vi "Clustering----.vi"() -> ()   [LabVIEW 2020]
panel:
  out "appended array":cluster{"array":dbl[], "array":dbl[]}[](array[cluster])
  in  "stop":bool
  out "byte swapped":u16
  out "Azimuth":u32
  out "100bytes":string
  out "Azimuth2":dbl
  out "substring 2":string
  in  "channel 1":bool=TRUE
  in  "channel 0":bool
  in  "channel 2":bool
  in  "channel 3":bool
  in  "channel 4":bool
  in  "channel 5":bool=TRUE
  in  "channel 6":bool
  in  "channel 7":bool
  in  "channel 8":bool
  in  "channel 9":bool
  in  "channel 10":bool
  in  "channel 11":bool
  in  "channel 12":bool
  in  "channel 13":bool
  in  "channel 14":bool
  in  "channel 15":bool
  in  "점 개수":i32
  out "Mixed Signal Graph":cluster{"array":dbl[], "array":dbl[]}[](graph)
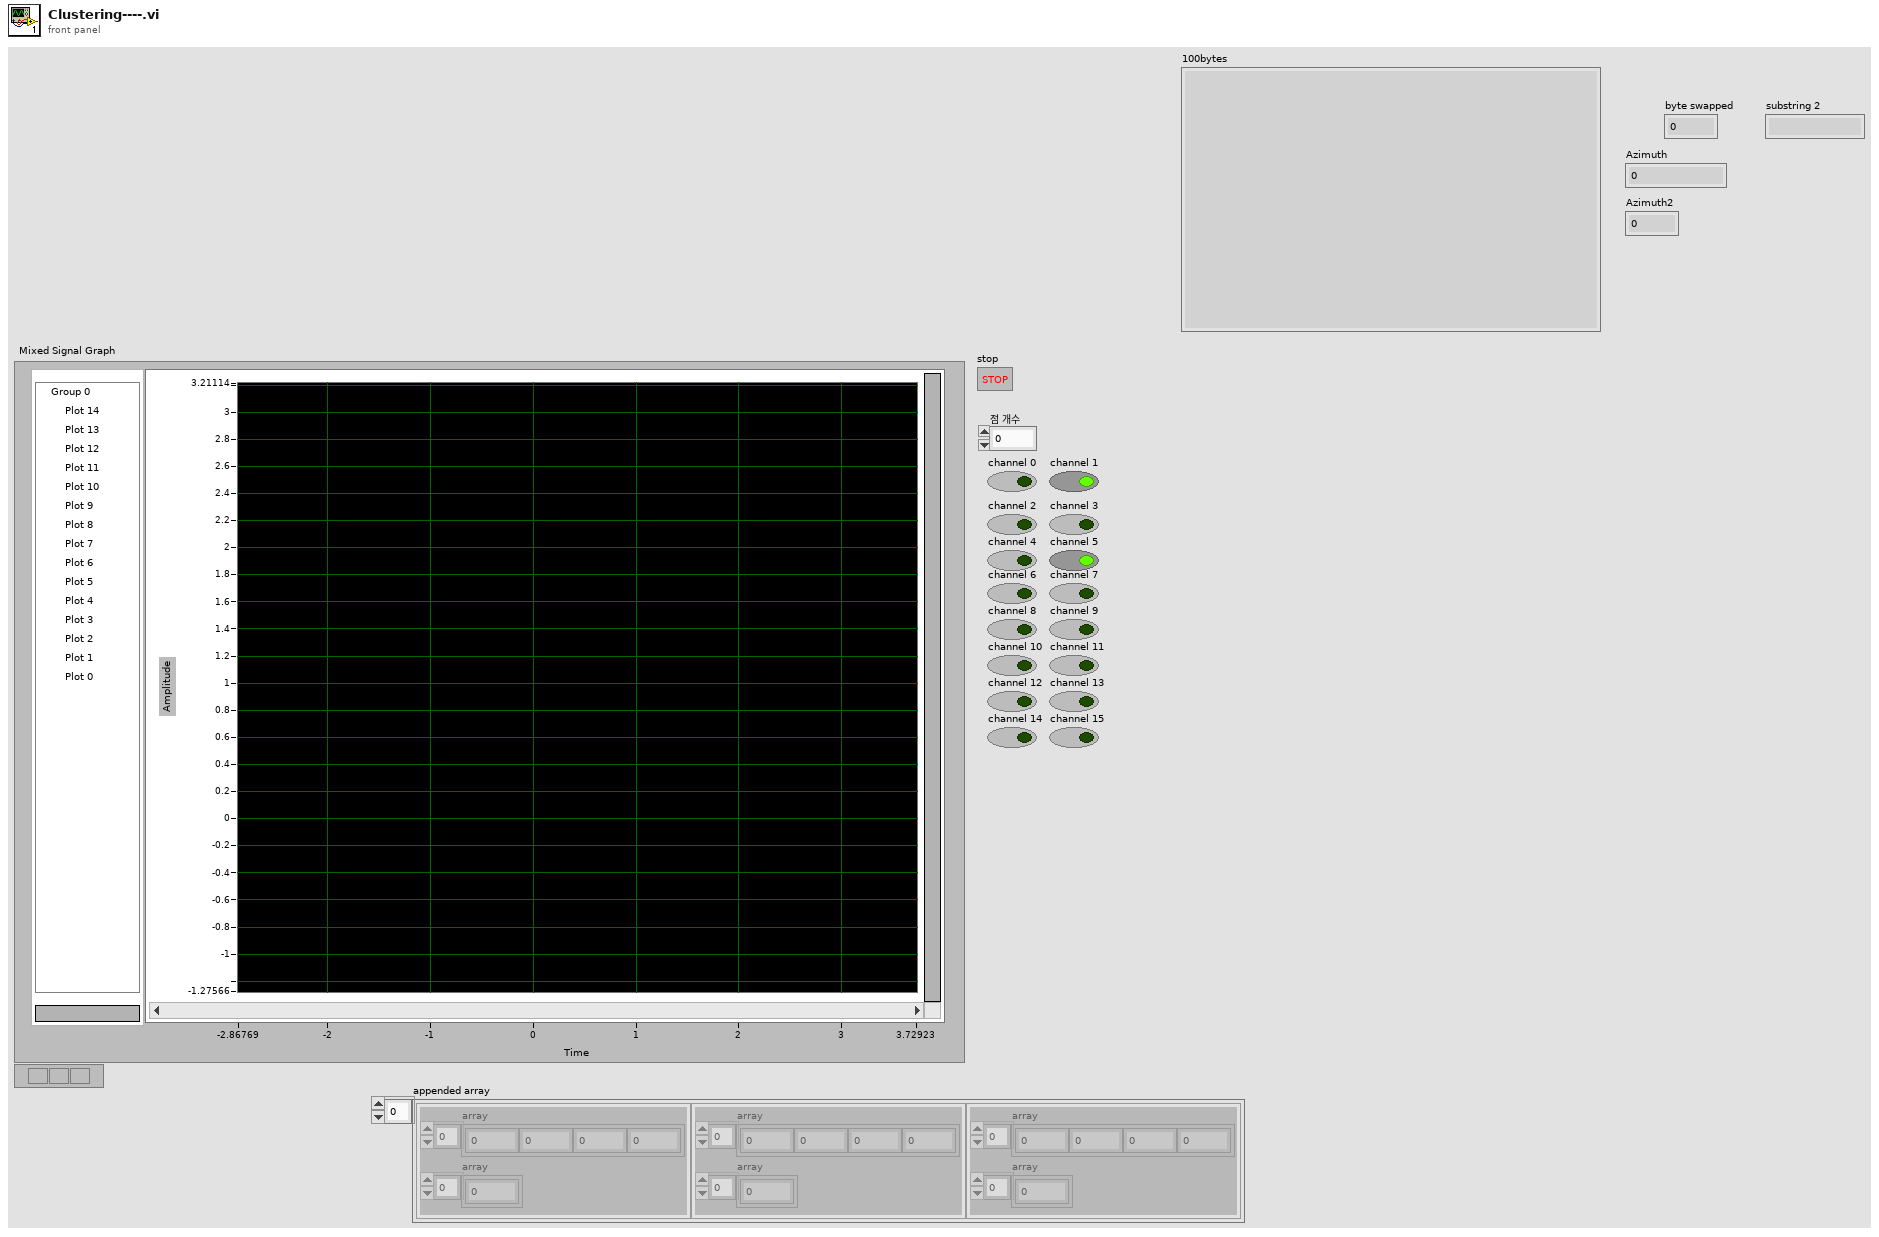
[diagram p1: front panel]
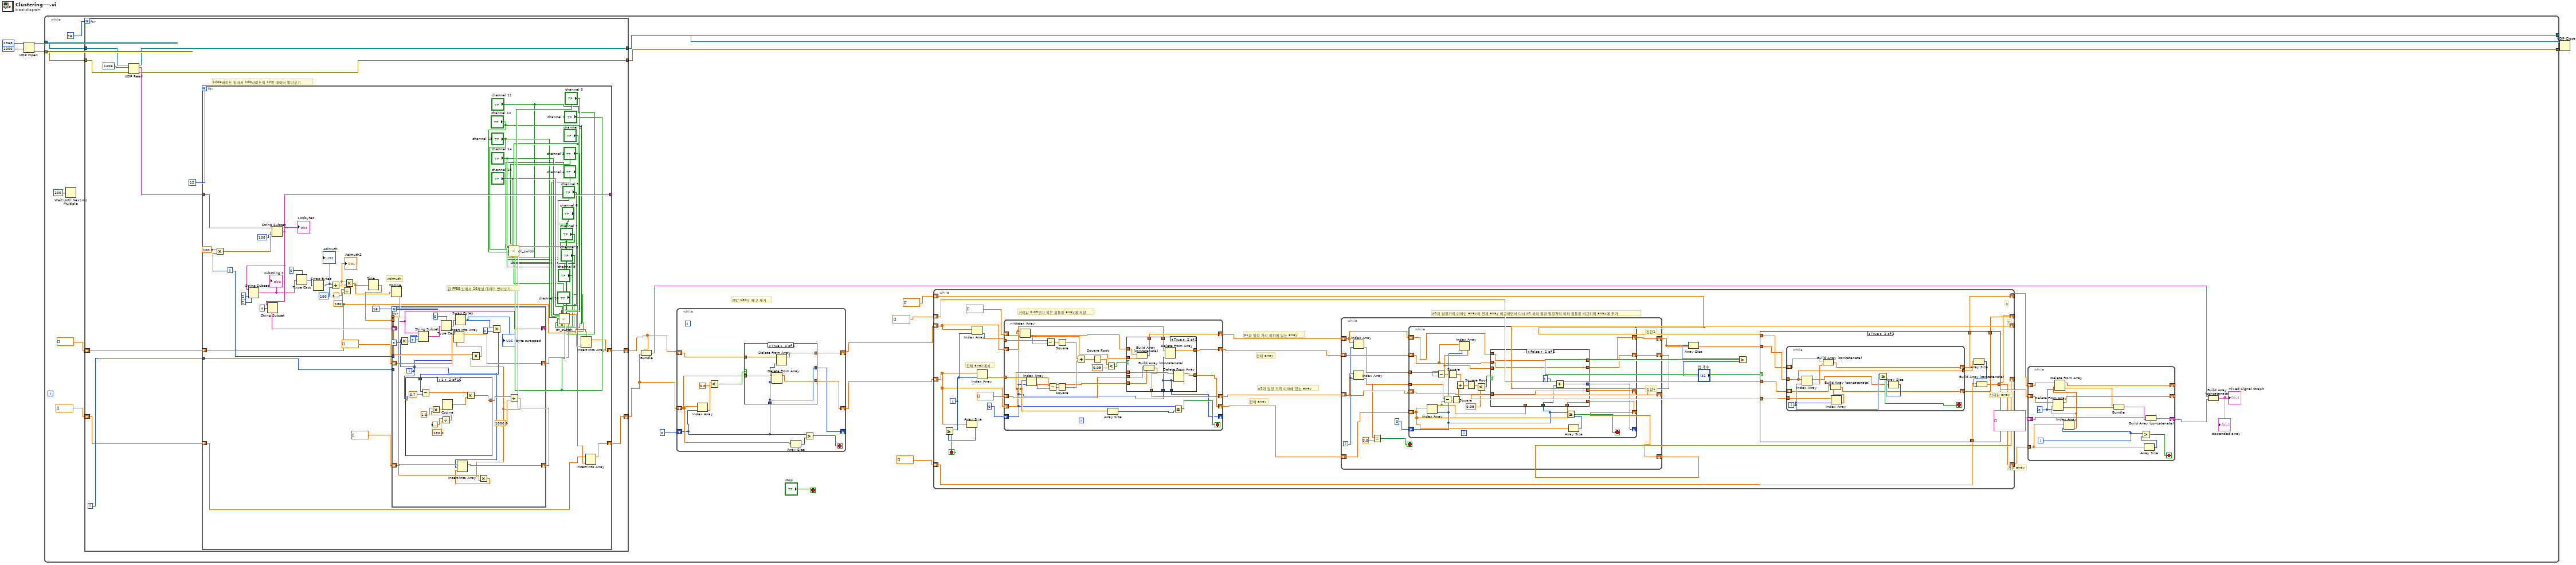
[diagram p0: block diagram]
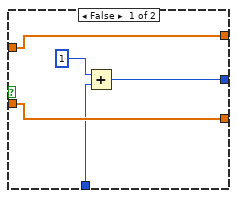
[diagram p2: hidden frame]
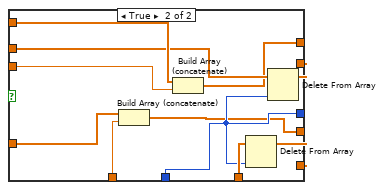
[diagram p4: hidden frame]
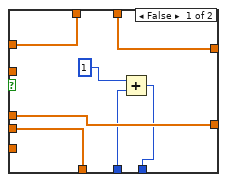
[diagram p5: hidden frame]
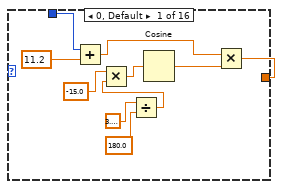
[diagram p6: hidden frame]
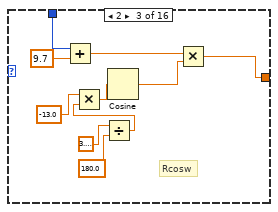
[diagram p7: hidden frame]
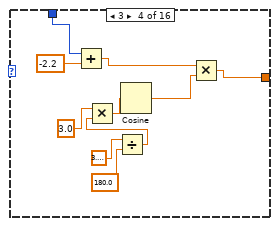
[diagram p8: hidden frame]
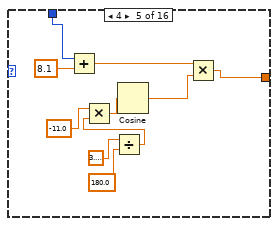
[diagram p9: hidden frame]
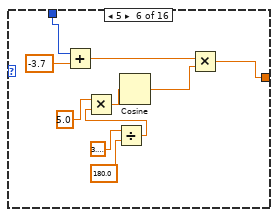
[diagram p10: hidden frame]
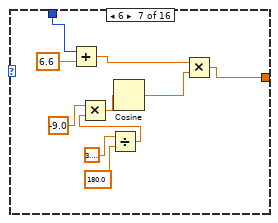
[diagram p11: hidden frame]
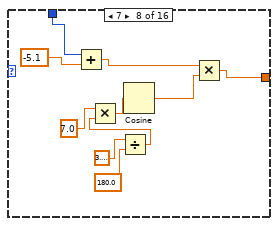
[diagram p12: hidden frame]
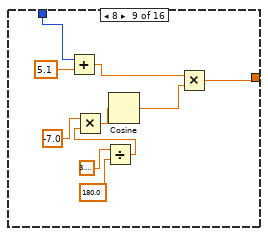
[diagram p13: hidden frame]
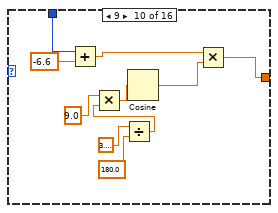
[diagram p14: hidden frame]
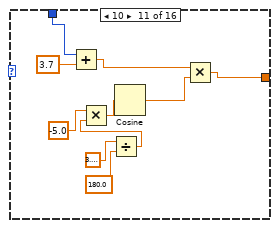
[diagram p15: hidden frame]
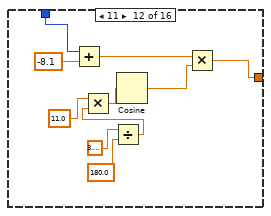
[diagram p16: hidden frame]
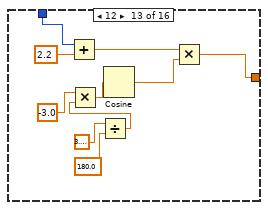
[diagram p17: hidden frame]
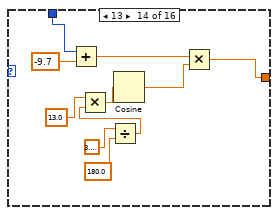
[diagram p18: hidden frame]
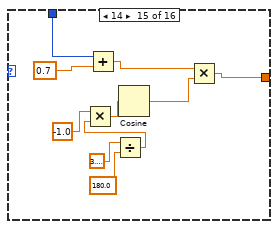
[diagram p19: hidden frame]
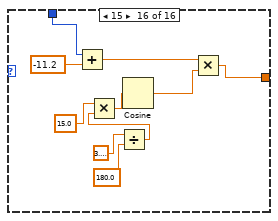
[diagram p20: hidden frame]
diagram:
  n1 = UDP Open(9:1000 ("timeout ms (25000)"), 11:u16 2368 ("port")) -> (port=w3:refnum<k16>, 0:w4:errorcluster)  [unwired: 3 in, 1 out]
  n2 = while {
    tunnel: w4 -> [w29]
    tunnel: w3 -> [w28]
    tunnel: [w27] -> w2
    tunnel: [w26] -> w1
    stop <- "stop" stop-if-true
    # "개수 array"
    # "Y"
    # "X"
    # "삭제된 array"
    # "전방 180도 빼고 제거"
    n3 = Wait Until Next ms Multiple(millisecond multiple=u32 100) -> ()  [unwired: 1 out]
    n4 = for {
      N: 76 -> [_]
      shift-right: [w218] -> w9
      shift-left: dbl[] [] ("array") -> [w216]
      shift-right: [w219] -> w10
      shift-left: dbl[] [] ("array") -> [w217]
      tunnel: w28 -> [w225]
      tunnel: [w222] -> w27
      tunnel: w29 -> [w226]
      tunnel: [w221] -> w26
      i -> [w220]
      # "1206바이트 읽어서 100바이트씩 12번 데이터 받아오기"
      n5 = UDP Read(connection ID=w225, max size (548)=1206, 8:w226) -> (data out=w224:string, error out=w221:errorcluster, 3:w222:refnum<k16>)  [unwired: 1 in, 2 out]
      n6 = for {
        N: 12 -> [_]
        shift-right: [w243] -> w218
        shift-left: w216 -> [w244]
        shift-right: [w246] -> w219
        shift-left: w217 -> [w248]
        tunnel: w220 -> [w255]
        tunnel: w224 -> [w263]
        tunnel: [w258] -> _
        i -> [w254]
        # "Azimuth"
        # "한 FFEE 안에서 16채널 데이터 받아오기"
        n7 = Multiply(x=100.0, y=w254) -> (x*y=w261:dbl)
        n8 = String Subset(string=w263, offset (0)=w261, length (rest)=100 ("length (rest)")) -> (substring=w258:string)
        "100bytes" <- w258
        n9 = String Subset(string=w258, offset (0)=2, length (rest)=2 ("length (rest)")) -> (substring=w257:string)
        "substring 2" <- w257
        n10 = String Subset(string=w258, offset (0)=4) -> (substring=w260:string)  [unwired: 1 in]
        n11 = Type Cast(type=u16 0, x=w257) -> (*(type *) &x=w256:u16)
        n12 = Swap Bytes(anything=w256) -> (byte swapped=w273:u16)
        "Azimuth" <- w273
        n13 = Divide(x=w273, y=u32 100) -> (x/y=w271:dbl)
        "Azimuth2" <- w271
        n14 = Divide(x=3.141592653589793, y=180.0) -> (x/y=w268:dbl)
        n15 = Multiply(x=w271, y=w268) -> (x*y=w266:dbl)
        n16 = Sine(x=w266) -> (sin(x)=w267:dbl)
        n17 = Cosine(x=w266) -> (cos(x)=w265:dbl)
        n18 = for {
          N: 16 -> [_]
          shift-right: [w295] -> w251
          shift-left: dbl[] [] ("array") -> [w296]
          tunnel: w267 -> [w289]
          shift-right: [w290] -> w253
          shift-left: dbl[] [] ("array") -> [w291]
          tunnel: w265 -> [w288]
          shift-right: [w283] -> _
          shift-left: w260 -> [w283]
          tunnel: w254 -> [_]
          tunnel: w255 -> [_]
          i -> [w278]
          n19 = Multiply(x=w278, y=3) -> (x*y=w297:i32)
          n20 = String Subset(string=w283, offset (0)=w297, length (rest)=2 ("length (rest)")) -> (substring=w285:string)
          n21 = Type Cast(type=u16 0, x=w285) -> (*(type *) &x=w284:u16)
          n22 = Swap Bytes(anything=w284) -> (byte swapped=w279:u16)
          "byte swapped" <- w279
          n23 = Multiply(x=w279, y=u32 2) -> (x*y=w293:u32)
          n24 = case shown="1" w278 {
            tunnel: w293 -> [w302 w312 w322 w331 w341 w351 w361 w371 w381 w391 w401 w411 w421 w431 w441 w451]
            tunnel: [w308 w313 w323 w333 w343 w353 w363 w373 w383 w393 w403 w413 w423 w433 w443 w453] -> w282
            frame 0, Default {
              n25 = Add(x=w302, y=11.2) -> (x+y=w300:dbl)
              n26 = Divide(x=3.141592653589793, y=180.0) -> (x/y=w303:dbl)
              n27 = Multiply(x=-15.0 ("y"), y=w303) -> (x*y=w304:dbl)
              n28 = Cosine(x=w304) -> (cos(x)=w309:dbl)
              n29 = Multiply(x=w300, y=w309) -> (x*y=w308:dbl)
            }
            frame 1 {
              n30 = Subtract(x=w312, y=0.7) -> (x-y=w310:dbl)
              n31 = Divide(x=3.141592653589793, y=180.0) -> (x/y=w315:dbl)
              n32 = Multiply(x=1.0 ("y"), y=w315) -> (x*y=w316:dbl)
              n33 = Cosine(x=w316) -> (cos(x)=w314:dbl)
              n34 = Multiply(x=w310, y=w314) -> (x*y=w313:dbl)
            }
            frame 2 {
              # "Rcosw"
              n35 = Add(x=w322, y=9.7) -> (x+y=w320:dbl)
              n36 = Divide(x=3.141592653589793, y=180.0) -> (x/y=w325:dbl)
              n37 = Multiply(x=-13.0 ("y"), y=w325) -> (x*y=w326:dbl)
              n38 = Cosine(x=w326) -> (cos(x)=w324:dbl)
              n39 = Multiply(x=w320, y=w324) -> (x*y=w323:dbl)
            }
            frame 3 {
              n40 = Add(x=w331, y=-2.2) -> (x+y=w330:dbl)
              n41 = Divide(x=3.141592653589793, y=180.0) -> (x/y=w335:dbl)
              n42 = Multiply(x=3.0 ("y"), y=w335) -> (x*y=w336:dbl)
              n43 = Cosine(x=w336) -> (cos(x)=w334:dbl)
              n44 = Multiply(x=w330, y=w334) -> (x*y=w333:dbl)
            }
            frame 4 {
              n45 = Add(x=w341, y=8.1) -> (x+y=w340:dbl)
              n46 = Divide(x=3.141592653589793, y=180.0) -> (x/y=w345:dbl)
              n47 = Multiply(x=-11.0 ("y"), y=w345) -> (x*y=w346:dbl)
              n48 = Cosine(x=w346) -> (cos(x)=w344:dbl)
              n49 = Multiply(x=w340, y=w344) -> (x*y=w343:dbl)
            }
            frame 5 {
              n50 = Add(x=w351, y=-3.7) -> (x+y=w350:dbl)
              n51 = Divide(x=3.141592653589793, y=180.0) -> (x/y=w355:dbl)
              n52 = Multiply(x=5.0 ("y"), y=w355) -> (x*y=w356:dbl)
              n53 = Cosine(x=w356) -> (cos(x)=w354:dbl)
              n54 = Multiply(x=w350, y=w354) -> (x*y=w353:dbl)
            }
            frame 6 {
              n55 = Add(x=w361, y=6.6) -> (x+y=w360:dbl)
              n56 = Divide(x=3.141592653589793, y=180.0) -> (x/y=w365:dbl)
              n57 = Multiply(x=-9.0 ("y"), y=w365) -> (x*y=w366:dbl)
              n58 = Cosine(x=w366) -> (cos(x)=w364:dbl)
              n59 = Multiply(x=w360, y=w364) -> (x*y=w363:dbl)
            }
            frame 7 {
              n60 = Add(x=w371, y=-5.1) -> (x+y=w370:dbl)
              n61 = Divide(x=3.141592653589793, y=180.0) -> (x/y=w375:dbl)
              n62 = Multiply(x=7.0 ("y"), y=w375) -> (x*y=w376:dbl)
              n63 = Cosine(x=w376) -> (cos(x)=w374:dbl)
              n64 = Multiply(x=w370, y=w374) -> (x*y=w373:dbl)
            }
            frame 8 {
              n65 = Add(x=w381, y=5.1) -> (x+y=w380:dbl)
              n66 = Divide(x=3.141592653589793, y=180.0) -> (x/y=w385:dbl)
              n67 = Multiply(x=-7.0 ("y"), y=w385) -> (x*y=w386:dbl)
              n68 = Cosine(x=w386) -> (cos(x)=w384:dbl)
              n69 = Multiply(x=w380, y=w384) -> (x*y=w383:dbl)
            }
            frame 9 {
              n70 = Add(x=w391, y=-6.6) -> (x+y=w390:dbl)
              n71 = Divide(x=3.141592653589793, y=180.0) -> (x/y=w395:dbl)
              n72 = Multiply(x=9.0 ("y"), y=w395) -> (x*y=w396:dbl)
              n73 = Cosine(x=w396) -> (cos(x)=w394:dbl)
              n74 = Multiply(x=w390, y=w394) -> (x*y=w393:dbl)
            }
            frame 10 {
              n75 = Add(x=w401, y=3.7) -> (x+y=w400:dbl)
              n76 = Divide(x=3.141592653589793, y=180.0) -> (x/y=w405:dbl)
              n77 = Multiply(x=-5.0 ("y"), y=w405) -> (x*y=w406:dbl)
              n78 = Cosine(x=w406) -> (cos(x)=w404:dbl)
              n79 = Multiply(x=w400, y=w404) -> (x*y=w403:dbl)
            }
            frame 11 {
              n80 = Add(x=w411, y=-8.1) -> (x+y=w410:dbl)
              n81 = Divide(x=3.141592653589793, y=180.0) -> (x/y=w415:dbl)
              n82 = Multiply(x=11.0 ("y"), y=w415) -> (x*y=w416:dbl)
              n83 = Cosine(x=w416) -> (cos(x)=w414:dbl)
              n84 = Multiply(x=w410, y=w414) -> (x*y=w413:dbl)
            }
            frame 12 {
              n85 = Add(x=w421, y=2.2) -> (x+y=w420:dbl)
              n86 = Divide(x=3.141592653589793, y=180.0) -> (x/y=w425:dbl)
              n87 = Multiply(x=-3.0 ("y"), y=w425) -> (x*y=w426:dbl)
              n88 = Cosine(x=w426) -> (cos(x)=w424:dbl)
              n89 = Multiply(x=w420, y=w424) -> (x*y=w423:dbl)
            }
            frame 13 {
              n90 = Add(x=w431, y=-9.7) -> (x+y=w430:dbl)
              n91 = Divide(x=3.141592653589793, y=180.0) -> (x/y=w435:dbl)
              n92 = Multiply(x=13.0 ("y"), y=w435) -> (x*y=w436:dbl)
              n93 = Cosine(x=w436) -> (cos(x)=w434:dbl)
              n94 = Multiply(x=w430, y=w434) -> (x*y=w433:dbl)
            }
            frame 14 {
              n95 = Add(x=w441, y=0.7) -> (x+y=w440:dbl)
              n96 = Divide(x=3.141592653589793, y=180.0) -> (x/y=w445:dbl)
              n97 = Multiply(x=-1.0 ("y"), y=w445) -> (x*y=w446:dbl)
              n98 = Cosine(x=w446) -> (cos(x)=w444:dbl)
              n99 = Multiply(x=w440, y=w444) -> (x*y=w443:dbl)
            }
            frame 15 {
              n100 = Add(x=w451, y=-11.2) -> (x+y=w450:dbl)
              n101 = Divide(x=3.141592653589793, y=180.0) -> (x/y=w455:dbl)
              n102 = Multiply(x=15.0 ("y"), y=w455) -> (x*y=w456:dbl)
              n103 = Cosine(x=w456) -> (cos(x)=w454:dbl)
              n104 = Multiply(x=w450, y=w454) -> (x*y=w453:dbl)
            }
          }
          n105 = Divide(x=w282, y=1000.0) -> (x/y=w280:dbl)
          n106 = Multiply(x=w289, y=w280) -> (x*y=w292:dbl)
          n107 = Insert Into Array(array=w296, index=w278, new element=w292) -> (w295:dbl[])
          n108 = Multiply(x=w280, y=w288) -> (x*y=w287:dbl)
          n109 = Insert Into Array(array=w291, index=w278, new element=w287) -> (w290:dbl[])
        }
        n110 = call "ch_switch.vi"("channel 14"="channel 14", "channel 4"="channel 4", "channel 13"="channel 13", "channel 5"="channel 5", "channel 12"="channel 12", "channel 6"="channel 6", "channel 7"="channel 7", "channel 3"="channel 3", "channel 8"="channel 8", "channel 15"="channel 15", "channel 9"="channel 9", "channel 2"="channel 2", "channel 10"="channel 10", "channel 1"="channel 1", "channel 11"="channel 11", "channel 0"="channel 0", "Array in"=w253) -> ("Array out"=w245:dbl[])  [unwired: 10 in]
        n111 = call "ch_switch.vi"("channel 14"="channel 14", "channel 4"="channel 4", "channel 13"="channel 13", "channel 5"="channel 5", "channel 12"="channel 12", "channel 6"="channel 6", "channel 7"="channel 7", "channel 3"="channel 3", "channel 8"="channel 8", "channel 15"="channel 15", "channel 9"="channel 9", "channel 2"="channel 2", "channel 10"="channel 10", "channel 1"="channel 1", "channel 11"="channel 11", "channel 0"="channel 0", "Array in"=w251) -> ("Array out"=w247:dbl[])  [unwired: 10 in]
        n112 = Insert Into Array(array=w248, new element=w247) -> (w246:dbl[])  [unwired: 1 in]
        n113 = Insert Into Array(array=w244, new element=w245) -> (w243:dbl[])  [unwired: 1 in]
      }
    }
    n114 = Bundle("array"=w10, "array"=w9) -> (w11:cluster{"array":dbl[], "array":dbl[]})  [unwired: 1 in]
    n115 = while {
      shift-right: [w51] -> w18
      shift-left: w9 -> [w50]
      shift-right: [w52] -> w22
      shift-left: w10 -> [w53]
      shift-right: [w46] -> _
      shift-left: 0 -> [w47]
      stop <- w48 stop-if-true
      n116 = Index Array(array=w50, index=w47) -> (element=w56:dbl)
      n117 = Less?(x=w56, y=0.0) -> (x < y?=w54:bool)
      n118 = case shown="True" w54 {
        tunnel: w53 -> [w61 w66]
        tunnel: w47 -> [w59 w62]
        tunnel: [w61 w63] -> w52
        tunnel: [w60 w64] -> w51
        tunnel: w50 -> [w60 w65]
        tunnel: [w58 w62] -> w46
        frame False {
          n119 = Add(x=1, y=w59) -> (x+y=w58:i32)
        }
        frame True {
          n120 = Delete From Array(array=w65, index=w62) -> (array with subset deleted=w64:dbl[])  [unwired: 1 in, 1 out]
          n121 = Delete From Array(array=w66, index=w62) -> (array with subset deleted=w63:dbl[])  [unwired: 1 in, 1 out]
        }
      }
      n122 = Array Size(array=w50) -> (size(s)=w49:i32)
      n123 = Greater?(x=w47, y=w49) -> (0:w48:bool)
    }
    n124 = while {
      shift-right: [w73] -> _
      shift-left: w22 -> [w83]
      shift-right: [w77] -> _
      shift-left: w18 -> [w82]
      shift-right: [w74] -> w12
      shift-left: dbl[] [] ("array") -> [w76]
      shift-right: [w70] -> w16
      shift-left: dbl[] [] ("array") -> [w75]
      shift-right: [w68] -> w15
      shift-left: dbl[] [] ("array") -> [w69]
      i -> [w91]
      stop <- w92 stop-if-true
      # "전체 array에서"
      # "전체 array"
      # "p1과 일정 거리 이하에 있는 array"
      # "전체 array"
      # "p1과 일정거리 이하인 array와 전체 array 비교하면서 다시 p1 외의 점과 일정거리 이하 점들을 비교하며 array에 추가"
      # "p1과 일정 거리 이하에 있는 array"
      # "거리값 0.05보다 작은 점들을 array에 저장"
      n125 = Array Size(array=w82) -> (size(s)=w93:i32)
      n126 = Greater Or Equal?(x=w91, y=w93) -> (x >= y?=w92:bool)
      n127 = Index Array(array=w83, index=w91) -> (element=w90:dbl)
      n128 = Index Array(array=w82, index=w91) -> (element=w89:dbl)
      n129 = while {
        tunnel: w90 -> [w197]
        tunnel: w89 -> [w196]
        shift-right: [w182] -> w71
        shift-left: dbl[] [] ("array") -> [w184]
        shift-right: [w183] -> w67
        shift-left: dbl[] [] ("array") -> [w185]
        shift-right: [w179] -> w78
        shift-left: w83 -> [w181]
        shift-right: [w178] -> w72
        shift-left: w82 -> [w180]
        shift-right: [w174] -> _
        shift-left: 0 -> [w175]
        stop <- w176 stop-if-true
        n130 = Index Array(array=w181, index=w175) -> (element=w187:dbl)
        n131 = Index Array(array=w180, index=w175) -> (element=w186:dbl)
        n132 = Subtract(x=w197, y=w187) -> (x-y=w195:dbl)
        n133 = Subtract(x=w196, y=w186) -> (x-y=w194:dbl)
        n134 = Square(x=w194) -> (x^2=w192:dbl)
        n135 = Square(x=w195) -> (x^2=w193:dbl)
        n136 = Add(x=w193, y=w192) -> (x+y=w191:dbl)
        n137 = Square Root(x=w191) -> (sqrt(x)=w190:dbl)
        n138 = Less?(x=w190, y=0.09) -> (x < y?=w188:bool)
        n139 = Array Size(array=w180) -> (size(s)=w177:i32)
        n140 = case shown="True" w188 {
          tunnel: w185 -> [w204 w212]
          tunnel: w184 -> [w203 w209]
          tunnel: w187 -> [_ w211]
          tunnel: w186 -> [_ w208]
          tunnel: [w204 w210] -> w183
          tunnel: [w203 w207] -> w182
          tunnel: w181 -> [w202 w215]
          tunnel: [w202 w206] -> w179
          tunnel: w180 -> [w201 w214]
          tunnel: [w201 w213] -> w178
          tunnel: w175 -> [w199 w205]
          tunnel: [w198 w205] -> w174
          frame False {
            n141 = Add(x=1, y=w199) -> (x+y=w198:i32)
          }
          frame True {
            n142 = Build Array (concatenate)(w212, w211) -> (w210:dbl[])
            n143 = Build Array (concatenate)(w209, w208) -> (w207:dbl[])
            n144 = Delete From Array(array=w215, index=w205) -> (array with subset deleted=w206:dbl[])  [unwired: 1 in, 1 out]
            n145 = Delete From Array(array=w214, index=w205) -> (array with subset deleted=w213:dbl[])  [unwired: 1 in, 1 out]
          }
        }
        n146 = Greater Or Equal?(x=w175, y=w177) -> (x >= y?=w176:bool)
      }
      n147 = while {
        shift-right: [w123] -> w80
        shift-left: w67 -> [w126]
        shift-right: [w129] -> w79
        shift-left: w71 -> [w128]
        shift-right: [w124] -> w73
        shift-left: w78 -> [w127]
        shift-right: [w130] -> w77
        shift-left: w72 -> [w122]
        i -> [w121]
        stop <- w118 stop-if-true
        # "집합1"
        # "집합1"
        n148 = Index Array(array=w128, index=w121) -> (element=w119:dbl)
        n149 = Index Array(array=w126, index=w121) -> (element=w125:dbl)
        n150 = Equal?(x=w119, y=0.0) -> (x = y?=w118:bool)
        n151 = while {
          tunnel: w125 -> [w155]
          tunnel: w119 -> [w154]
          shift-right: [w141] -> _
          shift-left: 0 -> [w142]
          shift-right: [w137] -> w129
          shift-left: w128 -> [w134]
          shift-right: [w133] -> w123
          shift-left: w126 -> [w140]
          shift-right: [w132] -> w124
          shift-left: w127 -> [w136]
          shift-right: [w139] -> w130
          shift-left: w122 -> [w138]
          stop <- w143 stop-if-true
          n152 = Index Array(array=w138, index=w142) -> (element=w135:dbl)
          n153 = Subtract(x=w154, y=w135) -> (x-y=w152:dbl)
          n154 = Square(x=w152) -> (x^2=w151:dbl)
          n155 = Index Array(array=w136, index=w142) -> (element=w145:dbl)
          n156 = Subtract(x=w155, y=w145) -> (x-y=w153:dbl)
          n157 = Square(x=w153) -> (x^2=w150:dbl)
          n158 = Add(x=w150, y=w151) -> (x+y=w149:dbl)
          n159 = Square Root(x=w149) -> (sqrt(x)=w148:dbl)
          n160 = Less?(x=w148, y=0.09) -> (x < y?=w146:bool)
          n161 = case shown="False" w146 {
            tunnel: w136 -> [w156 w165]
            tunnel: w142 -> [w161 w170]
            tunnel: w145 -> [_ w173]
            tunnel: [w157 w163] -> w133
            tunnel: w134 -> [w159 w172]
            tunnel: w140 -> [w157 w166]
            tunnel: w138 -> [w162 w171]
            tunnel: [w156 w167] -> w132
            tunnel: [w162 w168] -> w139
            tunnel: [w160 w170] -> w141
            tunnel: [w159 w169] -> w137
            tunnel: w135 -> [_ w164]
            frame False {
              n162 = Add(x=1, y=w161) -> (x+y=w160:i32)
            }
            frame True {
              n163 = Build Array (concatenate)(w172, w164) -> (w169:dbl[])
              n164 = Build Array (concatenate)(w166, w173) -> (w163:dbl[])
              n165 = Delete From Array(array=w171, index=w170) -> (array with subset deleted=w168:dbl[])  [unwired: 1 in, 1 out]
              n166 = Delete From Array(array=w165, index=w170) -> (array with subset deleted=w167:dbl[])  [unwired: 1 in, 1 out]
            }
          }
          n167 = Array Size(array=w138) -> (size(s)=w144:i32)
          n168 = Greater Or Equal?(x=w142, y=w144) -> (x >= y?=w143:bool)
        }
      }
      n169 = Array Size(array=w80) -> (size(s)=w85:i32)
      n170 = Greater?(x=w85, y="점 개수") -> (0:w86:bool)
      n171 = case shown="True" w86 {
        tunnel: w80 -> [_ w106]
        tunnel: w79 -> [_ w105]
        tunnel: w76 -> [w96 w104]
        tunnel: w75 -> [w95 w103]
        tunnel: [w96 w100] -> w74
        tunnel: [w95 w102] -> w70
        tunnel: w69 -> [w94 w99]
        tunnel: [w94 w98] -> w68
        frame False {
        }
        frame True {
          n172 = while {
            shift-right: [w109] -> w100
            shift-left: w104 -> [w112]
            tunnel: w106 -> [w107]
            shift-right: [w108] -> w102
            shift-left: w103 -> [w111]
            tunnel: w105 -> [w117]
            tunnel: [w107] -> w97
            i -> [w116]
            stop <- w114 stop-if-true
            n173 = Index Array(array=w107, index=w116) -> (element=w113:dbl)
            n174 = Build Array (concatenate)(w112, w113) -> (w109:dbl[])
            n175 = Index Array(array=w117, index=w116) -> (element=w110:dbl)
            n176 = Build Array (concatenate)(w111, w110) -> (w108:dbl[])
            n177 = Array Size(array=w107) -> (size(s)=w115:i32)
            n178 = Greater Or Equal?(x=w116, y=w115) -> (x >= y?=w114:bool)
          }
          n179 = Array Size(array=w97) -> (size(s)=w101:i32)
          n180 = Build Array (concatenate)(w99, w101) -> (w98:dbl[])
        }
      }
    }
    n181 = while {
      shift-right: [w40] -> _
      shift-left: w12 -> [w45]
      shift-right: [w37] -> _
      shift-left: w16 -> [w38]
      tunnel: w15 -> [w41]
      shift-right: [w33] -> w14
      shift-left: cluster{"array":dbl[], "array":dbl[]}[] [] -> [w32]
      i -> [w42]
      stop <- w43 stop-if-true
      w31 = 0 ("index")
      n182 = Index Array(array=w41, index=w42) -> (element=w39:dbl)
      n183 = Delete From Array(array=w38, length=w39, index=w31) -> (deleted portion=w35:dbl[], array with subset deleted=w37:dbl[])
      n184 = Delete From Array(array=w45, length=w39, index=w31) -> (deleted portion=w36:dbl[], array with subset deleted=w40:dbl[])
      n185 = Bundle("array"=w36, "array"=w35) -> (w34:cluster{"array":dbl[], "array":dbl[]})  [unwired: 1 in]
      n186 = Array Size(array=w41) -> (size(s)=w44:i32)
      n187 = Greater?(x=w42, y=w44) -> (0:w43:bool)
      n188 = Build Array (concatenate)(w32, w34) -> (w33:cluster{"array":dbl[], "array":dbl[]}[])
    }
    n189 = Build Array (concatenate)(w11, w14) -> (→"Mixed Signal Graph" →"appended array":cluster{"array":dbl[], "array":dbl[]}[])
  }
  n190 = UDP Close(connection ID=w2, 8:w1) -> ()  [unwired: 2 out]
